vi "move directory to protected Windows location.vi"(9 "Destination directory":path=path "C:/Program Files (x86)/National Instruments/RT Images/User Components", 10 "directory name (relative to system directory)":path=path "ProjectTemplates/Source/Linux Shared Memory and DCAF Example/cdf/Linux Shared Memory and DCAF", 11 "system directory (<LabVIEW>/vi.lib)":T1=14 items=["User Home", "User Desktop", "User Documents", "User Application Data", "User Preferences", "User Temporary", "Public Documents", "Public Application Data", "Public Preferences", "System Core Libraries", "System Installed Libraries", "Application Files", "Boot Volume Root", "Public Cache", "LabVIEW Default Directory", "LabVIEW Default Data", "LabVIEW VI Library", "Application Directory"]) -> (0 "error out":errorcluster, 1 "success?":bool, 2 "source directory":path)   [LabVIEW 2014]
uses:
  directory type.ctl
  <vilib>/Utility/sysdir.llb/System Directory Type.ctl
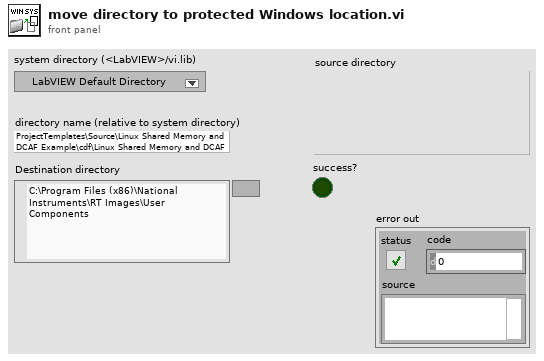
[diagram p1: front panel]
types:
  T1 = typedef "directory type.ctl" = i32
  T2 = typedef "System Directory Type.ctl" = i32
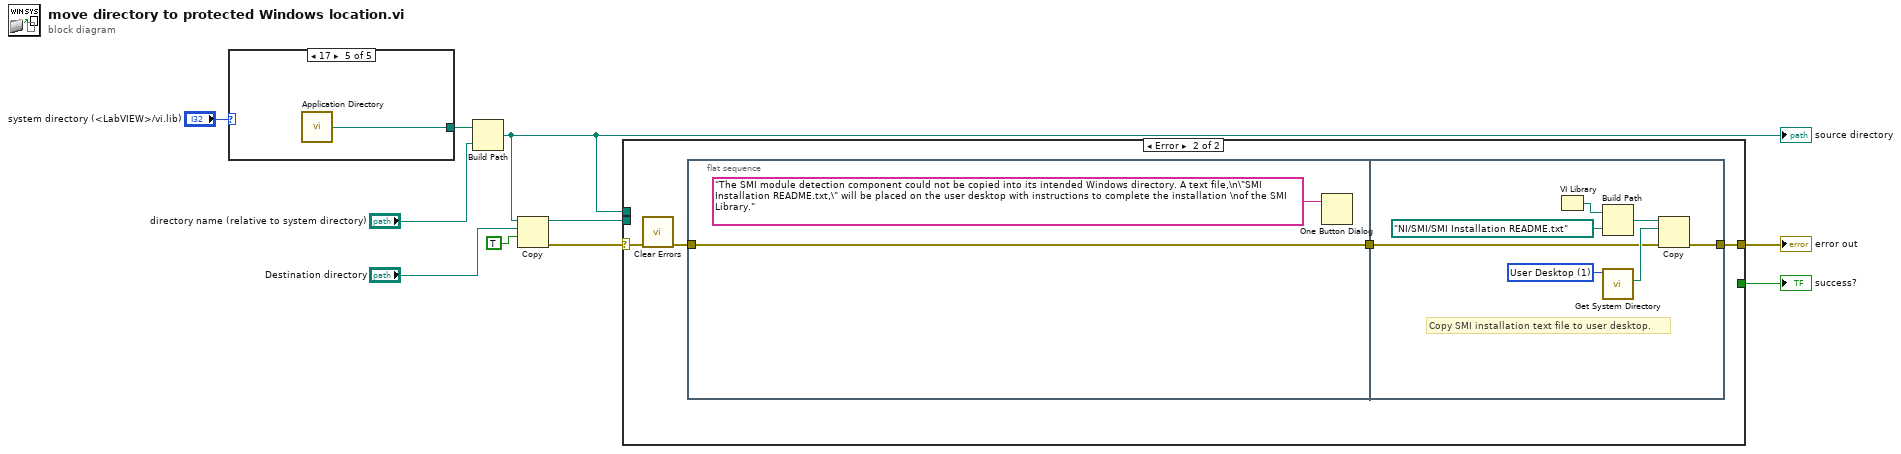
[diagram p0: block diagram]
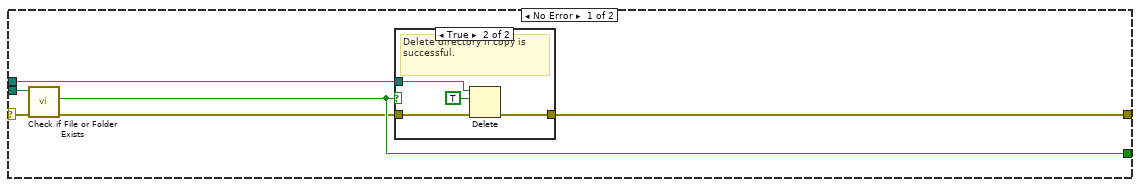
[diagram p2: hidden frame]
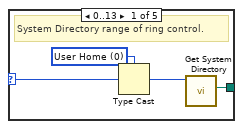
[diagram p4: hidden frame]
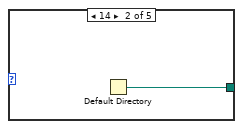
[diagram p5: hidden frame]
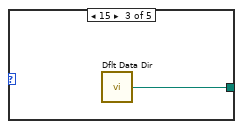
[diagram p6: hidden frame]
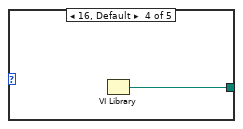
[diagram p7: hidden frame]
diagram:
  n1 = case shown="17" "system directory (<LabVIEW>/vi.lib)" {
    selector: "system directory (<LabVIEW>/vi.lib)" -> [w12 _ _ _ _]
    tunnel: [w14 w15 w16 w17 w18] -> w8
    frame 0..13 {
      w13 = T2 0 items=["User Home"=0, "User Desktop"=1, "User Documents"=2, "User Application Data"=3, "User Preferences"=4, "User Temporary"=5, "Public Documents"=6, "Public Application Data"=7, "Public Preferences"=8, "Public Cache"=13, "System Core Libraries"=9, "System Installed Libraries"=10, "Application Files"=11, "Boot Volume Root"=12] ("system directory type")
      # "System Directory range of ring control."
      n2 = Type Cast(type=w13, x=w12) -> (*(type *) &x=w11:T2)
      n3 = call <vilib>:"Get System Directory.vi"("system directory type"=w11) -> ("system directory"=w14:path)  [unwired: 10 in]
    }
    frame 14 {
      n4 = Default Directory() -> (w15:path)
    }
    frame 15 {
      n5 = call <vilib>:"Dflt Data Dir.vi"() -> ("App:Default Data Directory"=w16:path)
    }
    frame 16, Default {
      n6 = VI Library() -> (path=w17:path)
    }
    frame 17 {
      n7 = call <vilib>:"Application Directory.vi"() -> ("Application Directory"=w18:path)
    }
  }
  n8 = Build Path(base path=w8, name or relative path="directory name (relative to system directory)") -> (appended path=w1:path)
  "source directory" <- w1
  n9 = Copy(9:TRUE ("overwrite (F)"), 10:"Destination directory", 11:w1) -> (0:w2:errorcluster, 3:w3:path)  [unwired: 2 in, 1 out]
  n10 = case shown="Error" w2 {
    selector: w2 -> [w20 w33]
    tunnel: [w24 w31] -> w9
    tunnel: [w23 _] -> w6
    tunnel: w3 -> [w22 _]
    tunnel: w1 -> [w19 _]
    frame No Error {
      n11 = call <vilib>:"Check if File or Folder Exists.vi"("error in (no error)"=w20, "path"=w22) -> ("error out"=w21:errorcluster, "file or folder exists?"=w23:bool)  [unwired: 7 in, 1 out]
      n12 = case shown="True" w23 {
        tunnel: [w25 w29] -> w24
        tunnel: w19 -> [_ w28]
        tunnel: w21 -> [w25 w26]
        frame False {
        }
        frame True {
          # "Delete directory if copy is successful."
          n13 = Delete(path (use dialog)=w28, entire hierarchy (F)=TRUE, error in=w26) -> (error out=w29:errorcluster)  [unwired: 2 in, 2 out]
        }
      }
    }
    frame Error {
      n14 = call <vilib>:"Clear Errors.vi"("error in (no error)"=w33) -> ("error out"=w32:errorcluster)  [unwired: 5 in, 1 out]
      n15 = flat-sequence {
        tunnel: w32 -> [w35]
        tunnel: [w35] -> w30
        tunnel: [w36] -> w31
        tunnel: w30 -> [w37]
        frame #0 {
          n16 = One Button Dialog(message="The SMI module detection component could not be copied into its intended Windows directory. A text file,\n\"SMI Installation README.txt,\" will be placed on the user desktop with instructions to complete the installation \nof the SMI Library.") -> ()  [unwired: 1 in, 1 out]
        }
        frame #1 {
          w40 = T2 1 items=["User Home"=0, "User Desktop"=1, "User Documents"=2, "User Application Data"=3, "User Preferences"=4, "User Temporary"=5, "Public Documents"=6, "Public Application Data"=7, "Public Preferences"=8, "Public Cache"=13, "System Core Libraries"=9, "System Installed Libraries"=10, "Application Files"=11, "Boot Volume Root"=12] ("system directory type")
          # "Copy SMI installation text file to user desktop."
          n17 = VI Library() -> (path=w39:path)
          n18 = Build Path(base path=w39, name or relative path=path "NI/SMI/SMI Installation README.txt") -> (appended path=w41:path)
          n19 = call <vilib>:"Get System Directory.vi"("system directory type"=w40) -> ("system directory"=w42:path)  [unwired: 10 in]
          n20 = Copy(8:w37, 10:w42, 11:w41) -> (0:w36:errorcluster)  [unwired: 2 in, 2 out]
        }
      }
    }
  }
  "error out" <- w9
  "success?" <- w6
